vi "Begin Swerve Motors Brushless.vi"(2 "Steer Can Id":T2={"Front Left Steer CAN"=1, "Front Right Steer CAN"=1, "Back Left Steer CAN"=1, "Back Right Steer CAN"=1}, 3 "Drive Can Id":T1={"Front Left Drive CAN"=1, "Front Right Drive CAN"=1, "Back Left Drive CAN"=1, "Back Right Drive CAN"=1}) -> ()   [LabVIEW 2020]
uses:
  <vilib>/Rock Robotics/WPI/ThirdParty/REV Robotics/REVLib/Typedef/Spark MAX Limit Switch Polarity.ctl
  <vilib>/Rock Robotics/WPI/ThirdParty/REV Robotics/REVLib/Typedef/Spark MAX Limit Direction.ctl
  <vilib>/Rock Robotics/WPI/ThirdParty/REV Robotics/REVLib/Typedef/Spark MAX Motor Type.ctl
  <vilib>/Rock Robotics/WPI/ThirdParty/REV Robotics/REVLib/Typedef/Spark MAX Idle Mode.ctl
panel:
  in  "PID Constants Drive":T3={"P Gain"=2.5e-10, "I Gain"=0.0, "D Gain"=0.0, "F Gain"=0.000175, "I Zone"=0.0, "Min Output"=-1.0, "Max Output"=1.0} {"P Gain" format="%#_9f"}
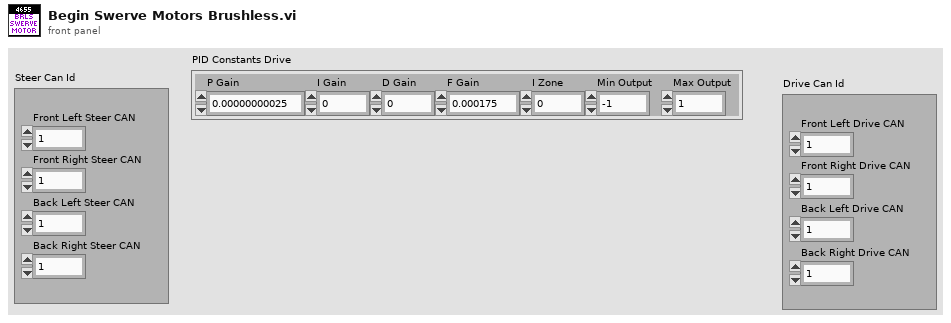
[diagram p1: front panel]
types:
  T1 = cluster{"Front Left Drive CAN":u8, "Front Right Drive CAN":u8, "Back Left Drive CAN":u8, "Back Right Drive CAN":u8}
  T2 = cluster{"Front Left Steer CAN":u8, "Front Right Steer CAN":u8, "Back Left Steer CAN":u8, "Back Right Steer CAN":u8}
  T3 = cluster{"P Gain":dbl, "I Gain":dbl, "D Gain":dbl, "F Gain":dbl, "I Zone":dbl, "Min Output":dbl, "Max Output":dbl}
  T4 = typedef "Spark MAX Idle Mode.ctl" = enum16{"Coast", "Brake"}
  T5 = typedef "Spark MAX Limit Direction.ctl" = enum16{"Forward Limit", "Reverse Limit"}
  T6 = typedef "Spark MAX Limit Switch Polarity.ctl" = enum16{"Normally Open", "Normally Closed"}
  T7 = typedef "Spark MAX Motor Type.ctl" = enum16{"Brushed", "Brushless"}
  T8 = typedef "WPI_MotorControlDeviceRef.ctl" = cluster{"DeviceStatus":errorcluster, "Type":T9, "PWM":cluster{"PWM Channel":T10, "DeadBand":T11}, "CAN":cluster{"Device Number":u8, "SetOutput VI Ref":variant, "GetOutput VI Ref":variant, "Enable VI Ref":variant, "Disable VI Ref":variant, "Data":variant}, "Invert":bool, "DIO PWM":cluster{"PWM \"Enable\" Channel":T10, "DIOChannel":T12, "PWM Rate":dbl}}
  T9 = typedef "WPI_MotorControlType.ctl" = enum16{"PWM", "CAN", "DIO PWM"}
  T10 = typedef "FPGA_DIOPWMChannel.ctl" = enum8{"PWM 0", "PWM 1", "PWM 2", "PWM 3", "PWM 4", "PWM 5", "PWM 6", "PWM 7", "PWM 8", "PWM 9", "PWM MXP 0", "PWM MXP 1", "PWM MXP 2", "PWM MXP 3", "PWM MXP 4", "PWM MXP 5", "PWM MXP 6", "PWM MXP 7", "PWM MXP 8", "PWM MXP 9", "Invalid"}
  T11 = typedef "WPI_PWMDeadband.ctl" = cluster{"Name":string, "maxPositivePwm":i32, "minPositivePwm":i32, "centerPwm":i32, "maxNegativePwm":i32, "minNegativePwm":i32, "angularRange":u16}
  T12 = typedef "FPGA_DIOChannel.ctl" = enum8{"DIO 0", "DIO 1", "DIO 2", "DIO 3", "DIO 4", "DIO 5", "DIO 6", "DIO 7", "DIO 8", "DIO 9", "DIO MXP 0", "DIO MXP 1", "DIO MXP 2", "DIO MXP 3", "DIO MXP 4", "DIO MXP 5", "DIO MXP 6", "DIO MXP 7", "DIO MXP 8", "DIO MXP 9", "DIO MXP 10", "DIO MXP 11", "DIO MXP 12", "DIO MXP 13", "DIO MXP 14", "DIO MXP 15", "SPI Port CS1", "SPI Port CS2", "SPI Port CS3", "SPI Port MISO", "SPI Port MOSI", "Invalid"}
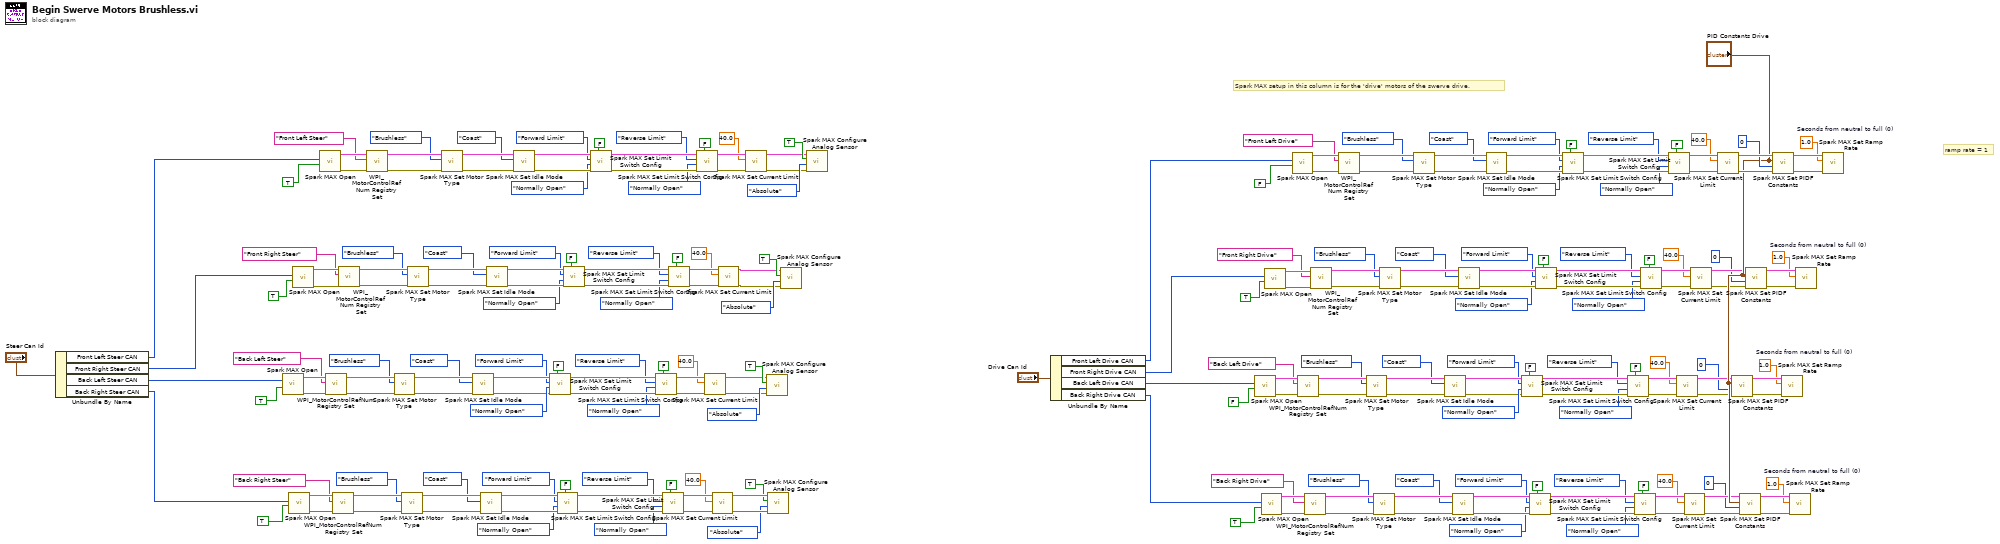
[diagram p0: block diagram]
diagram:
  w15 = sgl 1.0  # Seconds from neutral to full (0)
  w38 = sgl 1.0  # Seconds from neutral to full (0)
  w65 = sgl 1.0  # Seconds from neutral to full (0)
  w221 = sgl 1.0  # Seconds from neutral to full (0)
  # "ramp rate = 1"
  # "Spark MAX setup in this column is for the 'drive' motors of the swerve drive."
  n1 = Unbundle By Name("Steer Can Id") -> ("Front Left Steer CAN"=w176:u8, "Front Right Steer CAN"=w177:u8, "Back Left Steer CAN"=w178:u8, "Back Right Steer CAN"=w179:u8)
  n2 = call <vilib>:"Spark MAX Open.vi"("Invert"=TRUE, "Device Number"=w178) -> ("error out"=w120:errorcluster, "MotorControlDeviceRef"=w121:T8)  [unwired: 8 in]
  n3 = call <vilib>:"Spark MAX Open.vi"("Invert"=TRUE, "Device Number"=w179) -> ("error out"=w162:errorcluster, "MotorControlDeviceRef"=w163:T8)  [unwired: 8 in]
  n4 = call <vilib>:"Spark MAX Open.vi"("Invert"=TRUE, "Device Number"=w177) -> ("error out"=w140:errorcluster, "MotorControlDeviceRef"=w141:T8)  [unwired: 8 in]
  n5 = call <vilib>:"Spark MAX Open.vi"("Invert"=TRUE, "Device Number"=w176) -> ("error out"=w181:errorcluster, "MotorControlDeviceRef"=w182:T8)  [unwired: 8 in]
  n6 = call <vilib>:"WPI_MotorControlRefNum Registry Set.vi"("error in (no error)"=w120, "refnum name"="Back Left Steer" ("Motor References"), "MotorControlDevRef"=w121) -> ("error out"=w135:errorcluster, "MotorControlDevRef"=w136:T8)  [unwired: 7 in]
  n7 = call <vilib>:"WPI_MotorControlRefNum Registry Set.vi"("error in (no error)"=w162, "refnum name"="Back Right Steer" ("Motor References"), "MotorControlDevRef"=w163) -> ("error out"=w167:errorcluster, "MotorControlDevRef"=w168:T8)  [unwired: 7 in]
  n8 = call <vilib>:"WPI_MotorControlRefNum Registry Set.vi"("error in (no error)"=w140, "refnum name"="Front Right Steer" ("Motor References"), "MotorControlDevRef"=w141) -> ("error out"=w157:errorcluster, "MotorControlDevRef"=w158:T8)  [unwired: 7 in]
  n9 = call <vilib>:"WPI_MotorControlRefNum Registry Set.vi"("error in (no error)"=w181, "refnum name"="Front Left Steer" ("Motor References"), "MotorControlDevRef"=w182) -> ("error out"=w198:errorcluster, "MotorControlDevRef"=w199:T8)  [unwired: 7 in]
  n10 = call <vilib>:"Spark MAX Set Motor Type.vi"("error in (no error)"=w135, "Motor Type"=Spark_MAX_Motor_Type."Brushless" ("Enum"), "MotorControlDevRef"=w136) -> ("error out"=w133:errorcluster, "MotorControlDeviceRef"=w134:T8)  [unwired: 7 in]
  n11 = call <vilib>:"Spark MAX Set Motor Type.vi"("error in (no error)"=w167, "Motor Type"=Spark_MAX_Motor_Type."Brushless" ("Enum"), "MotorControlDevRef"=w168) -> ("error out"=w165:errorcluster, "MotorControlDeviceRef"=w166:T8)  [unwired: 7 in]
  n12 = call <vilib>:"Spark MAX Set Motor Type.vi"("error in (no error)"=w157, "Motor Type"=Spark_MAX_Motor_Type."Brushless" ("Enum"), "MotorControlDevRef"=w158) -> ("error out"=w155:errorcluster, "MotorControlDeviceRef"=w156:T8)  [unwired: 7 in]
  n13 = call <vilib>:"Spark MAX Set Motor Type.vi"("error in (no error)"=w198, "Motor Type"=Spark_MAX_Motor_Type."Brushless" ("Enum"), "MotorControlDevRef"=w199) -> ("error out"=w196:errorcluster, "MotorControlDeviceRef"=w197:T8)  [unwired: 7 in]
  n14 = call <vilib>:"Spark MAX Set Idle Mode.vi"("error in (no error)"=w133, "Idle Mode"=Spark_MAX_Idle_Mode."Coast", "MotorControlDeviceRef in"=w134) -> ("error out"=w103:errorcluster, "MotorControlDeviceRef out"=w132:T8)  [unwired: 7 in]
  n15 = call <vilib>:"Spark MAX Set Idle Mode.vi"("error in (no error)"=w165, "Idle Mode"=Spark_MAX_Idle_Mode."Coast", "MotorControlDeviceRef in"=w166) -> ("error out"=w115:errorcluster, "MotorControlDeviceRef out"=w116:T8)  [unwired: 7 in]
  n16 = call <vilib>:"Spark MAX Set Idle Mode.vi"("error in (no error)"=w155, "Idle Mode"=Spark_MAX_Idle_Mode."Coast", "MotorControlDeviceRef in"=w156) -> ("error out"=w153:errorcluster, "MotorControlDeviceRef out"=w154:T8)  [unwired: 7 in]
  n17 = call <vilib>:"Spark MAX Set Idle Mode.vi"("error in (no error)"=w196, "Idle Mode"=Spark_MAX_Idle_Mode."Coast", "MotorControlDeviceRef in"=w197) -> ("error out"=w194:errorcluster, "MotorControlDeviceRef out"=w195:T8)  [unwired: 7 in]
  n18 = call <vilib>:"Spark MAX Set Limit Switch Config.vi"("Enabled? (T)"=FALSE, "error in (no error)"=w103, "Polarity (Normally Open)"=Spark_MAX_Limit_Switch_Polarity."Normally Open", "Limit Switch"=Spark_MAX_Limit_Direction."Forward Limit", "MotorControlDeviceRef in"=w132) -> ("error out"=w130:errorcluster, "MotorControlDeviceRef out"=w131:T8)  [unwired: 5 in]
  n19 = call <vilib>:"Spark MAX Set Limit Switch Config.vi"("Enabled? (T)"=FALSE, "error in (no error)"=w115, "Polarity (Normally Open)"=Spark_MAX_Limit_Switch_Polarity."Normally Open", "Limit Switch"=Spark_MAX_Limit_Direction."Forward Limit", "MotorControlDeviceRef in"=w116) -> ("error out"=w113:errorcluster, "MotorControlDeviceRef out"=w114:T8)  [unwired: 5 in]
  n20 = call <vilib>:"Spark MAX Set Limit Switch Config.vi"("Enabled? (T)"=FALSE, "error in (no error)"=w153, "Polarity (Normally Open)"=Spark_MAX_Limit_Switch_Polarity."Normally Open", "Limit Switch"=Spark_MAX_Limit_Direction."Forward Limit", "MotorControlDeviceRef in"=w154) -> ("error out"=w151:errorcluster, "MotorControlDeviceRef out"=w152:T8)  [unwired: 5 in]
  n21 = call <vilib>:"Spark MAX Set Limit Switch Config.vi"("Enabled? (T)"=FALSE, "error in (no error)"=w194, "Polarity (Normally Open)"=Spark_MAX_Limit_Switch_Polarity."Normally Open", "Limit Switch"=Spark_MAX_Limit_Direction."Forward Limit", "MotorControlDeviceRef in"=w195) -> ("error out"=w192:errorcluster, "MotorControlDeviceRef out"=w193:T8)  [unwired: 5 in]
  n22 = call <vilib>:"Spark MAX Set Limit Switch Config.vi"("Enabled? (T)"=FALSE, "error in (no error)"=w130, "Polarity (Normally Open)"=Spark_MAX_Limit_Switch_Polarity."Normally Open", "Limit Switch"=Spark_MAX_Limit_Direction."Reverse Limit", "MotorControlDeviceRef in"=w131) -> ("error out"=w138:errorcluster, "MotorControlDeviceRef out"=w137:T8)  [unwired: 5 in]
  n23 = call <vilib>:"Spark MAX Set Limit Switch Config.vi"("Enabled? (T)"=FALSE, "error in (no error)"=w113, "Polarity (Normally Open)"=Spark_MAX_Limit_Switch_Polarity."Normally Open", "Limit Switch"=Spark_MAX_Limit_Direction."Reverse Limit", "MotorControlDeviceRef in"=w114) -> ("error out"=w118:errorcluster, "MotorControlDeviceRef out"=w117:T8)  [unwired: 5 in]
  n24 = call <vilib>:"Spark MAX Set Limit Switch Config.vi"("Enabled? (T)"=FALSE, "error in (no error)"=w151, "Polarity (Normally Open)"=Spark_MAX_Limit_Switch_Polarity."Normally Open", "Limit Switch"=Spark_MAX_Limit_Direction."Reverse Limit", "MotorControlDeviceRef in"=w152) -> ("error out"=w160:errorcluster, "MotorControlDeviceRef out"=w159:T8)  [unwired: 5 in]
  n25 = call <vilib>:"Spark MAX Set Limit Switch Config.vi"("Enabled? (T)"=FALSE, "error in (no error)"=w192, "Polarity (Normally Open)"=Spark_MAX_Limit_Switch_Polarity."Normally Open", "Limit Switch"=Spark_MAX_Limit_Direction."Reverse Limit", "MotorControlDeviceRef in"=w193) -> ("error out"=w201:errorcluster, "MotorControlDeviceRef out"=w200:T8)  [unwired: 5 in]
  n26 = call <vilib>:"Spark MAX Set Current Limit.vi"("error in (no error)"=w138, "Current Limit A (100)"=sgl 40.0, "MotorControlDeviceRef in"=w137) -> ("error out"=w88:errorcluster, "MotorControlDeviceRef out"=w89:T8)  [unwired: 7 in]
  n27 = call <vilib>:"Spark MAX Set Current Limit.vi"("error in (no error)"=w118, "Current Limit A (100)"=sgl 40.0, "MotorControlDeviceRef in"=w117) -> ("error out"=w99:errorcluster, "MotorControlDeviceRef out"=w98:T8)  [unwired: 7 in]
  n28 = call <vilib>:"Spark MAX Set Current Limit.vi"("error in (no error)"=w160, "Current Limit A (100)"=sgl 40.0, "MotorControlDeviceRef in"=w159) -> ("error out"=w90:errorcluster, "MotorControlDeviceRef out"=w91:T8)  [unwired: 7 in]
  n29 = call <vilib>:"Spark MAX Set Current Limit.vi"("error in (no error)"=w201, "Current Limit A (100)"=sgl 40.0, "MotorControlDeviceRef in"=w200) -> ("error out"=w169:errorcluster, "MotorControlDeviceRef out"=w170:T8)  [unwired: 7 in]
  n30 = call <vilib>:"Spark MAX Configure Analog Sensor.vi"("error in (no error)"=w88, "Sensor Mode (Absolute)"=enum16{"Absolute", "Relative"}."Absolute", "Inverted (F)"=TRUE, "MotorControlDeviceRef in"=w89) -> ()  [unwired: 6 in, 2 out]
  n31 = call <vilib>:"Spark MAX Configure Analog Sensor.vi"("error in (no error)"=w99, "Sensor Mode (Absolute)"=enum16{"Absolute", "Relative"}."Absolute", "Inverted (F)"=TRUE, "MotorControlDeviceRef in"=w98) -> ()  [unwired: 6 in, 2 out]
  n32 = call <vilib>:"Spark MAX Configure Analog Sensor.vi"("error in (no error)"=w90, "Sensor Mode (Absolute)"=enum16{"Absolute", "Relative"}."Absolute", "Inverted (F)"=TRUE, "MotorControlDeviceRef in"=w91) -> ()  [unwired: 6 in, 2 out]
  n33 = call <vilib>:"Spark MAX Configure Analog Sensor.vi"("error in (no error)"=w169, "Sensor Mode (Absolute)"=enum16{"Absolute", "Relative"}."Absolute", "Inverted (F)"=TRUE, "MotorControlDeviceRef in"=w170) -> ()  [unwired: 6 in, 2 out]
  n34 = Unbundle By Name("Drive Can Id") -> ("Front Left Drive CAN"=w205:u8, "Front Right Drive CAN"=w202:u8, "Back Left Drive CAN"=w203:u8, "Back Right Drive CAN"=w204:u8)
  n35 = call <vilib>:"Spark MAX Open.vi"("Invert"=FALSE, "Device Number"=w203) -> ("error out"=w27:errorcluster, "MotorControlDeviceRef"=w28:T8)  [unwired: 8 in]
  n36 = call <vilib>:"Spark MAX Open.vi"("Invert"=TRUE, "Device Number"=w204) -> ("error out"=w81:errorcluster, "MotorControlDeviceRef"=w82:T8)  [unwired: 8 in]
  n37 = call <vilib>:"Spark MAX Open.vi"("Invert"=TRUE, "Device Number"=w202) -> ("error out"=w53:errorcluster, "MotorControlDeviceRef"=w54:T8)  [unwired: 8 in]
  n38 = call <vilib>:"Spark MAX Open.vi"("Invert"=FALSE, "Device Number"=w205) -> ("error out"=w209:errorcluster, "MotorControlDeviceRef"=w210:T8)  [unwired: 8 in]
  n39 = call <vilib>:"WPI_MotorControlRefNum Registry Set.vi"("error in (no error)"=w27, "refnum name"="Back Left Drive" ("Motor References"), "MotorControlDevRef"=w28) -> ("error out"=w48:errorcluster, "MotorControlDevRef"=w49:T8)  [unwired: 7 in]
  n40 = call <vilib>:"WPI_MotorControlRefNum Registry Set.vi"("error in (no error)"=w81, "refnum name"="Back Right Drive" ("Motor References"), "MotorControlDevRef"=w82) -> ("error out"=w86:errorcluster, "MotorControlDevRef"=w87:T8)  [unwired: 7 in]
  n41 = call <vilib>:"WPI_MotorControlRefNum Registry Set.vi"("error in (no error)"=w53, "refnum name"="Front Right Drive" ("Motor References"), "MotorControlDevRef"=w54) -> ("error out"=w76:errorcluster, "MotorControlDevRef"=w77:T8)  [unwired: 7 in]
  n42 = call <vilib>:"WPI_MotorControlRefNum Registry Set.vi"("error in (no error)"=w209, "refnum name"="Front Left Drive" ("Motor References"), "MotorControlDevRef"=w210) -> ("error out"=w232:errorcluster, "MotorControlDevRef"=w233:T8)  [unwired: 7 in]
  n43 = call <vilib>:"Spark MAX Set Motor Type.vi"("error in (no error)"=w48, "Motor Type"=Spark_MAX_Motor_Type."Brushless" ("Enum"), "MotorControlDevRef"=w49) -> ("error out"=w46:errorcluster, "MotorControlDeviceRef"=w47:T8)  [unwired: 7 in]
  n44 = call <vilib>:"Spark MAX Set Motor Type.vi"("error in (no error)"=w86, "Motor Type"=Spark_MAX_Motor_Type."Brushless" ("Enum"), "MotorControlDevRef"=w87) -> ("error out"=w84:errorcluster, "MotorControlDeviceRef"=w85:T8)  [unwired: 7 in]
  n45 = call <vilib>:"Spark MAX Set Motor Type.vi"("error in (no error)"=w76, "Motor Type"=Spark_MAX_Motor_Type."Brushless" ("Enum"), "MotorControlDevRef"=w77) -> ("error out"=w74:errorcluster, "MotorControlDeviceRef"=w75:T8)  [unwired: 7 in]
  n46 = call <vilib>:"Spark MAX Set Motor Type.vi"("error in (no error)"=w232, "Motor Type"=Spark_MAX_Motor_Type."Brushless" ("Enum"), "MotorControlDevRef"=w233) -> ("error out"=w230:errorcluster, "MotorControlDeviceRef"=w231:T8)  [unwired: 7 in]
  n47 = call <vilib>:"Spark MAX Set Idle Mode.vi"("error in (no error)"=w46, "Idle Mode"=Spark_MAX_Idle_Mode."Coast", "MotorControlDeviceRef in"=w47) -> ("error out"=w4:errorcluster, "MotorControlDeviceRef out"=w45:T8)  [unwired: 7 in]
  n48 = call <vilib>:"Spark MAX Set Idle Mode.vi"("error in (no error)"=w84, "Idle Mode"=Spark_MAX_Idle_Mode."Coast", "MotorControlDeviceRef in"=w85) -> ("error out"=w22:errorcluster, "MotorControlDeviceRef out"=w23:T8)  [unwired: 7 in]
  n49 = call <vilib>:"Spark MAX Set Idle Mode.vi"("error in (no error)"=w74, "Idle Mode"=Spark_MAX_Idle_Mode."Coast", "MotorControlDeviceRef in"=w75) -> ("error out"=w72:errorcluster, "MotorControlDeviceRef out"=w73:T8)  [unwired: 7 in]
  n50 = call <vilib>:"Spark MAX Set Idle Mode.vi"("error in (no error)"=w230, "Idle Mode"=Spark_MAX_Idle_Mode."Coast", "MotorControlDeviceRef in"=w231) -> ("error out"=w228:errorcluster, "MotorControlDeviceRef out"=w229:T8)  [unwired: 7 in]
  n51 = call <vilib>:"Spark MAX Set Limit Switch Config.vi"("Enabled? (T)"=FALSE, "error in (no error)"=w4, "Polarity (Normally Open)"=Spark_MAX_Limit_Switch_Polarity."Normally Open", "Limit Switch"=Spark_MAX_Limit_Direction."Forward Limit", "MotorControlDeviceRef in"=w45) -> ("error out"=w43:errorcluster, "MotorControlDeviceRef out"=w44:T8)  [unwired: 5 in]
  n52 = call <vilib>:"Spark MAX Set Limit Switch Config.vi"("Enabled? (T)"=FALSE, "error in (no error)"=w22, "Polarity (Normally Open)"=Spark_MAX_Limit_Switch_Polarity."Normally Open", "Limit Switch"=Spark_MAX_Limit_Direction."Forward Limit", "MotorControlDeviceRef in"=w23) -> ("error out"=w20:errorcluster, "MotorControlDeviceRef out"=w21:T8)  [unwired: 5 in]
  n53 = call <vilib>:"Spark MAX Set Limit Switch Config.vi"("Enabled? (T)"=FALSE, "error in (no error)"=w72, "Polarity (Normally Open)"=Spark_MAX_Limit_Switch_Polarity."Normally Open", "Limit Switch"=Spark_MAX_Limit_Direction."Forward Limit", "MotorControlDeviceRef in"=w73) -> ("error out"=w70:errorcluster, "MotorControlDeviceRef out"=w71:T8)  [unwired: 5 in]
  n54 = call <vilib>:"Spark MAX Set Limit Switch Config.vi"("Enabled? (T)"=FALSE, "error in (no error)"=w228, "Polarity (Normally Open)"=Spark_MAX_Limit_Switch_Polarity."Normally Open", "Limit Switch"=Spark_MAX_Limit_Direction."Forward Limit", "MotorControlDeviceRef in"=w229) -> ("error out"=w226:errorcluster, "MotorControlDeviceRef out"=w227:T8)  [unwired: 5 in]
  n55 = call <vilib>:"Spark MAX Set Limit Switch Config.vi"("Enabled? (T)"=FALSE, "error in (no error)"=w43, "Polarity (Normally Open)"=Spark_MAX_Limit_Switch_Polarity."Normally Open", "Limit Switch"=Spark_MAX_Limit_Direction."Reverse Limit", "MotorControlDeviceRef in"=w44) -> ("error out"=w51:errorcluster, "MotorControlDeviceRef out"=w50:T8)  [unwired: 5 in]
  n56 = call <vilib>:"Spark MAX Set Limit Switch Config.vi"("Enabled? (T)"=FALSE, "error in (no error)"=w20, "Polarity (Normally Open)"=Spark_MAX_Limit_Switch_Polarity."Normally Open", "Limit Switch"=Spark_MAX_Limit_Direction."Reverse Limit", "MotorControlDeviceRef in"=w21) -> ("error out"=w25:errorcluster, "MotorControlDeviceRef out"=w24:T8)  [unwired: 5 in]
  n57 = call <vilib>:"Spark MAX Set Limit Switch Config.vi"("Enabled? (T)"=FALSE, "error in (no error)"=w70, "Polarity (Normally Open)"=Spark_MAX_Limit_Switch_Polarity."Normally Open", "Limit Switch"=Spark_MAX_Limit_Direction."Reverse Limit", "MotorControlDeviceRef in"=w71) -> ("error out"=w79:errorcluster, "MotorControlDeviceRef out"=w78:T8)  [unwired: 5 in]
  n58 = call <vilib>:"Spark MAX Set Limit Switch Config.vi"("Enabled? (T)"=FALSE, "error in (no error)"=w226, "Polarity (Normally Open)"=Spark_MAX_Limit_Switch_Polarity."Normally Open", "Limit Switch"=Spark_MAX_Limit_Direction."Reverse Limit", "MotorControlDeviceRef in"=w227) -> ("error out"=w235:errorcluster, "MotorControlDeviceRef out"=w234:T8)  [unwired: 5 in]
  n59 = call <vilib>:"Spark MAX Set Current Limit.vi"("error in (no error)"=w51, "Current Limit A (100)"=sgl 40.0, "MotorControlDeviceRef in"=w50) -> ("error out"=w41:errorcluster, "MotorControlDeviceRef out"=w42:T8)  [unwired: 7 in]
  n60 = call <vilib>:"Spark MAX Set Current Limit.vi"("error in (no error)"=w25, "Current Limit A (100)"=sgl 40.0, "MotorControlDeviceRef in"=w24) -> ("error out"=w18:errorcluster, "MotorControlDeviceRef out"=w19:T8)  [unwired: 7 in]
  n61 = call <vilib>:"Spark MAX Set Current Limit.vi"("error in (no error)"=w79, "Current Limit A (100)"=sgl 40.0, "MotorControlDeviceRef in"=w78) -> ("error out"=w68:errorcluster, "MotorControlDeviceRef out"=w69:T8)  [unwired: 7 in]
  n62 = call <vilib>:"Spark MAX Set Current Limit.vi"("error in (no error)"=w235, "Current Limit A (100)"=sgl 40.0, "MotorControlDeviceRef in"=w234) -> ("error out"=w224:errorcluster, "MotorControlDeviceRef out"=w225:T8)  [unwired: 7 in]
  n63 = call <vilib>:"Spark MAX Set PIDF Constants.vi"("error in"=w41, "PIDF Slot"=0, "PID Constants"="PID Constants Drive", "MotorControlDeviceRef"=w42) -> ("error out"=w39:errorcluster, "MotorControlDeviceRef"=w40:T8)  [unwired: 6 in]
  n64 = call <vilib>:"Spark MAX Set PIDF Constants.vi"("error in"=w18, "PIDF Slot"=0, "PID Constants"="PID Constants Drive", "MotorControlDeviceRef"=w19) -> ("error out"=w16:errorcluster, "MotorControlDeviceRef"=w17:T8)  [unwired: 6 in]
  n65 = call <vilib>:"Spark MAX Set PIDF Constants.vi"("error in"=w68, "PIDF Slot"=0, "PID Constants"="PID Constants Drive", "MotorControlDeviceRef"=w69) -> ("error out"=w66:errorcluster, "MotorControlDeviceRef"=w67:T8)  [unwired: 6 in]
  n66 = call <vilib>:"Spark MAX Set PIDF Constants.vi"("error in"=w224, "PIDF Slot"=0, "PID Constants"="PID Constants Drive", "MotorControlDeviceRef"=w225) -> ("error out"=w222:errorcluster, "MotorControlDeviceRef"=w223:T8)  [unwired: 6 in]
  n67 = call <vilib>:"Spark MAX Set Ramp Rate.vi"("error in (no error)"=w39, "Seconds from neutral to full (0)"=w38, "MotorControlDeviceRef in"=w40) -> ()  [unwired: 7 in, 2 out]
  n68 = call <vilib>:"Spark MAX Set Ramp Rate.vi"("error in (no error)"=w16, "Seconds from neutral to full (0)"=w15, "MotorControlDeviceRef in"=w17) -> ()  [unwired: 7 in, 2 out]
  n69 = call <vilib>:"Spark MAX Set Ramp Rate.vi"("error in (no error)"=w66, "Seconds from neutral to full (0)"=w65, "MotorControlDeviceRef in"=w67) -> ()  [unwired: 7 in, 2 out]
  n70 = call <vilib>:"Spark MAX Set Ramp Rate.vi"("error in (no error)"=w222, "Seconds from neutral to full (0)"=w221, "MotorControlDeviceRef in"=w223) -> ()  [unwired: 7 in, 2 out]
